vi "EnableStageAcquire.vi"(8 "error in (no error)":errorcluster, 11 "Microscope in":refnum<class "Microscope.lvclass">) -> (0 "error out":errorcluster, 3 "Microscope out":refnum<class "Microscope.lvclass">)   [LabVIEW 2012, in "Microscope.lvclass"]
uses:
  classes/Microscope.lvclass
  typedefs/Move Type.ctl
  classes/Microscope.lvclass/Microscope.ctl
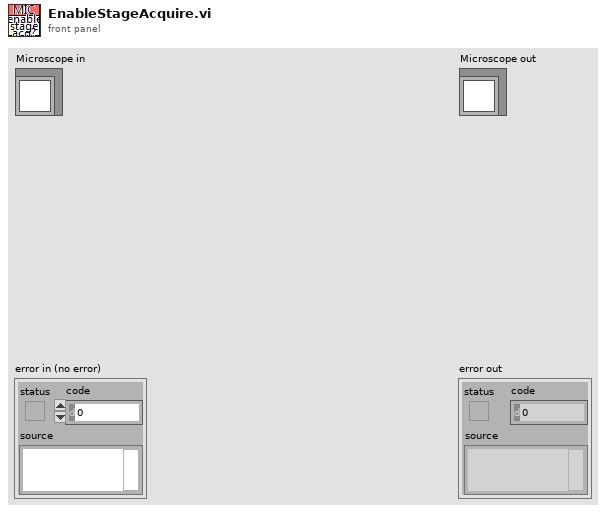
[diagram p1: front panel]
types:
  T1 = typedef "Move Type.ctl" = enum16{"None", "Continuous", "Discrete"}
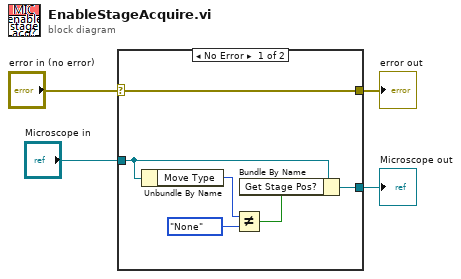
[diagram p0: block diagram]
diagram:
  n1 = case shown="No Error" "error in (no error)" {
    selector: "error in (no error)" -> [w10 w12]
    tunnel: [w10 w12] -> w3
    tunnel: [w6 w11] -> w1
    tunnel: "Microscope in" -> [w7 w11]
    frame No Error {
      n2 = Unbundle By Name(w7) -> ("Move Type"=w9:T1)
      n3 = Not Equal?(x=w9, y=Move_Type."None") -> (x != y?=w5:bool)
      n4 = Bundle By Name(cluster=w7, "Get Stage Pos?"=w5) -> (w6:refnum<class "Microscope.lvclass">)
    }
    frame Error {
    }
  }
  "error out" <- w3
  "Microscope out" <- w1
